vi "Example_QueryFmt.vi"(3 "supported by":enum16{"Device", "Mixer"}(ring)=enum."Mixer", 4 "Format":cluster{"Rate":i32, "Bits":i32, "Channels":i32}={"Rate"=44100, "Bits"=16, "Channels"=2}, 5 "use WASAPI":bool, 6 "Direction (Record)":u16(ring) items=["Record", "Play"], 7 "idev":u32) -> (0 "error out":errorcluster, 1 "Conf":i32[](array[numeric])=[48000, 16, 1, 0])   [LabVIEW 2016]
uses:
  WaveIO.dll
panel:
  in  "channel Mask?":bool
  # "Samples/s"
  # "Bits/sample"
  # "# channels"
  # "channel mask"
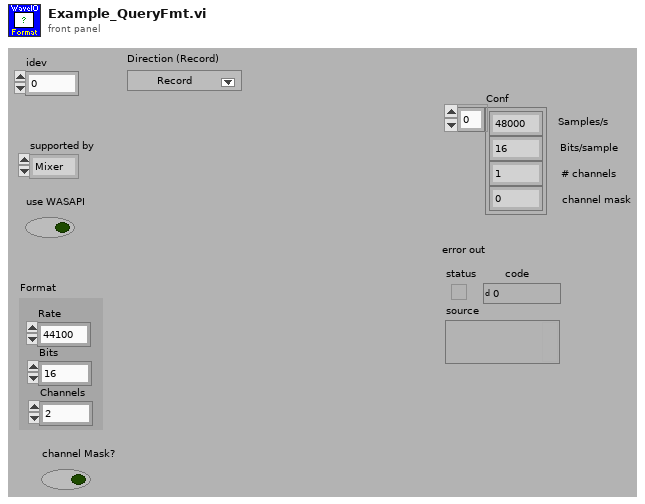
[diagram p1: front panel]
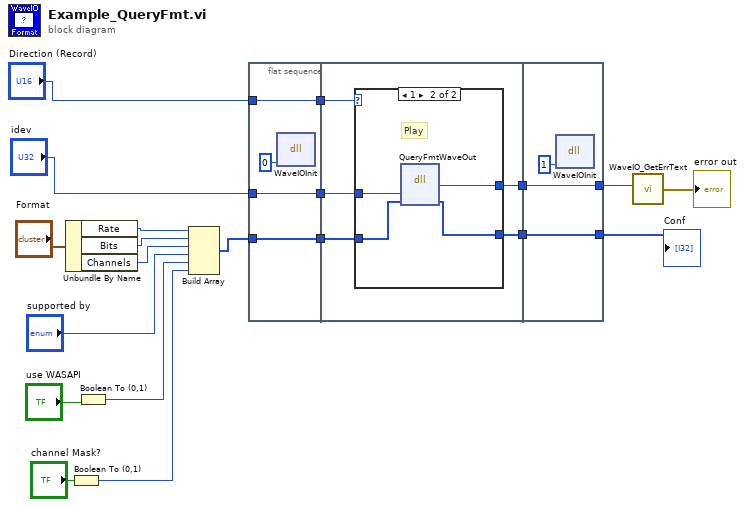
[diagram p0: block diagram]
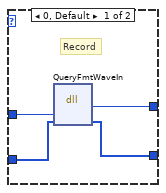
[diagram p2: hidden frame]
diagram:
  n1 = Unbundle By Name("Format") -> ("Rate"=w16:i32, "Bits"=w15:i32, "Channels"=w14:i32)
  n2 = Boolean To (0,1)(Boolean="channel Mask?") -> (0, 1=w6:i16)
  n3 = Boolean To (0,1)(Boolean="use WASAPI") -> (0, 1=w8:i16)
  n4 = Build Array(w16, w15, w14, "supported by", w8, w6) -> (w13:i32[])
  n5 = flat-sequence {
    tunnel: w13 -> [w22]
    tunnel: "Direction (Record)" -> [w23]
    tunnel: "idev" -> [w24]
    tunnel: [w24] -> w5
    tunnel: [w23] -> w4
    tunnel: [w22] -> w3
    tunnel: w5 -> [w29]
    tunnel: w4 -> [w27]
    tunnel: w3 -> [w26]
    tunnel: [w28] -> w2
    tunnel: [w25] -> w1
    tunnel: [w39] -> w10
    tunnel: [w40] -> w19
    tunnel: w2 -> [w40]
    tunnel: w1 -> [w39]
    frame #0 {
      n6 = dll-call lib="D:/Dokumenty/Uczelnia/LabVIEW 2/Lab2 - 09.10.2018/WaveIO/waveio.dll" fn="WaveIOInit"("flag"=0) -> ()  [unwired: 5 in, 2 out]
    }
    frame #1 {
      n7 = case shown="1" w27 {
        tunnel: w29 -> [w32 w37]
        tunnel: [w33 w36] -> w28
        tunnel: w26 -> [w31 w35]
        tunnel: [w30 w34] -> w25
        frame 0, Default {
          # "Record"
          n8 = dll-call lib="D:/Dokumenty/Uczelnia/LabVIEW 2/Lab2 - 09.10.2018/WaveIO/waveio.dll" fn="QueryFmtWaveIn"("iDev"=w32, "Conf"=w31) -> (w33:i32, "Conf"=w30:i32[])  [unwired: 4 in, 2 out]
        }
        frame 1 {
          # "Play"
          n9 = dll-call lib="D:/Dokumenty/Uczelnia/LabVIEW 2/Lab2 - 09.10.2018/WaveIO/waveio.dll" fn="QueryFmtWaveOut"("idev"=w37, "Conf"=w35) -> (w36:i32, "Conf"=w34:i32[])  [unwired: 4 in, 2 out]
        }
      }
    }
    frame #2 {
      n10 = dll-call lib="D:/Dokumenty/Uczelnia/LabVIEW 2/Lab2 - 09.10.2018/WaveIO/waveio.dll" fn="WaveIOInit"("flag"=1) -> ()  [unwired: 5 in, 2 out]
    }
  }
  n11 = call "WaveIO_GetErrText.vi"("ErrorCode"=w19) -> ("error out"=→"error out":errorcluster)
  "Conf" <- w10
